vi "Spreadsheet name number.vi"(8 "error in":errorcluster, 9 "Terminal String":string, 10 "Numbers":dbl[](array[numeric]), 11 "Names":string[](array[string])) -> (0 "error out":errorcluster, 3 "Spreadsheet String":string)   [LabVIEW 2019]
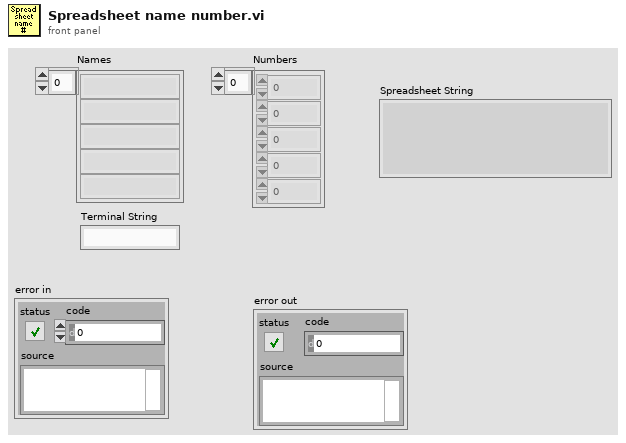
[diagram p1: front panel]
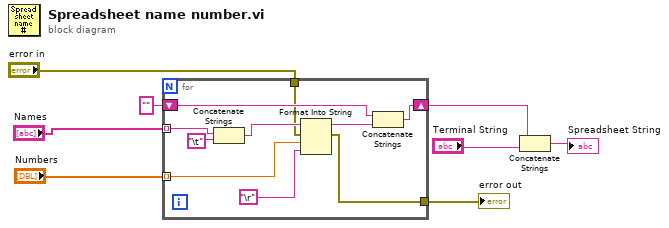
[diagram p0: block diagram]
diagram:
  n1 = for {
    tunnel: "Names" -> [w18] mode=indexing
    tunnel: "Numbers" -> [w16] mode=indexing
    shift-right: [w13] -> w4
    shift-left: "" -> [w12]
    tunnel: [w10] -> w6
    tunnel: "error in" -> [w9]
    n2 = Concatenate Strings(w18, "\t") -> (w15:string)
    n3 = Format Into String(initial string=w15, error in=w9, w16, "\r") -> (resulting string=w11:string, error out=w10:errorcluster)  [unwired: 1 in]
    n4 = Concatenate Strings(w12, w11) -> (w13:string)
  }
  "error out" <- w6
  n5 = Concatenate Strings(w4, "Terminal String") -> (→"Spreadsheet String":string)
